vi "Remote.vi"() -> ()   [LabVIEW 2020]
uses:
  LMH-PS4/Private/Type Defs/Indicators/Controller.ctl
  LMH-PS4/Private/Type Defs/Indicators/Square.ctl
  LMH-PS4/Private/Type Defs/Indicators/X.ctl
  LMH-PS4/Private/Type Defs/Indicators/Circle.ctl
  LMH-PS4/Private/Type Defs/Indicators/Triangle.ctl
  LMH-PS4/Private/Type Defs/Indicators/L1.ctl
  LMH-PS4/Private/Type Defs/Indicators/R1.ctl
  LMH-PS4/Private/Type Defs/Indicators/Share.ctl
  LMH-PS4/Private/Type Defs/Indicators/Options.ctl
  LMH-PS4/Private/Type Defs/Indicators/PS.ctl
  LMH-PS4/Private/Type Defs/Indicators/Pad_Button.ctl
  LMH-PS4/Private/Type Defs/Indicators/Dpad.ctl
  LMH-PS4/Private/Type Defs/Indicators/Slider.ctl
  <vilib>/Platform/TimedLoop/XDataNode/timing_clust.ctl
  <vilib>/Platform/TimedLoop/XDataNode/nitl_modes.ctl
  <vilib>/Platform/TimedLoop/XDataNode/wakeup.ctl
  <vilib>/CISH Robotics/L4VMX VMXpi/Type Def/VMX Channel Index.ctl
  <vilib>/CISH Robotics/L4VMX TitanQuad/Motor ID.ctl
  <vilib>/CISH Robotics/L4VMX TitanQuad/TitanQuad.lvclass
  <vilib>/CISH Robotics/L4VMX VMXpi/PWM Generator/PWM Generator.lvclass
  <vilib>/platform/TimedLoop/XDataNode/XDataNode.xnode
  <vilib>/ReMiSYS Technology/RemoteToolkit/Receiver/Receiver.lvclass
  LMH-PS4/LMH-PS4.lvlib
  <vilib>/CISH Robotics/L4VMX VMXpi/Power/Power.lvclass
  <vilib>/Platform/TimedLoop/XDataNode/XDNodeRunTimeDep.lvlib
  <vilib>/CISH Robotics/L4VMX VMXpi/L4VMX.lvlib
  <vilib>/CISH Robotics/L4VMX VMXpi/Utilities/Utilities.lvclass
  <vilib>/CISH Robotics/L4VMX VMXpi/Digital Output/Digital Output.lvclass
  <vilib>/CISH Robotics/L4VMX VMXpi/Digital Input/Digital Input.lvclass
panel:
  out "x/y":dbl
  out "Stop0":bool
  out "result":dbl[](array[numeric])
  out "Voltage":sgl
  out "Error Out":errorcluster
  in  "Stop":bool
  out "Received?":bool
  out "PS4 Controller":T1={"Square Button"=FALSE, "X Button"=FALSE, "Circle Button"=FALSE, "Triangle Button"=FALSE, "L1"=FALSE, "R1"=FALSE, "Share Button"=FALSE, "Options Button"=FALSE, "PS Button"=FALSE, "Pad Button"=FALSE, "D-Pad"=5, "L2"=0, "R2"=0, "Thumbstick_Left"={[], []}, "Thumbstick_Right"={[], []}} {"R2" scale=-32768.0..32767.0; "L2" scale=-32768.0..32767.0}
  # "ss"
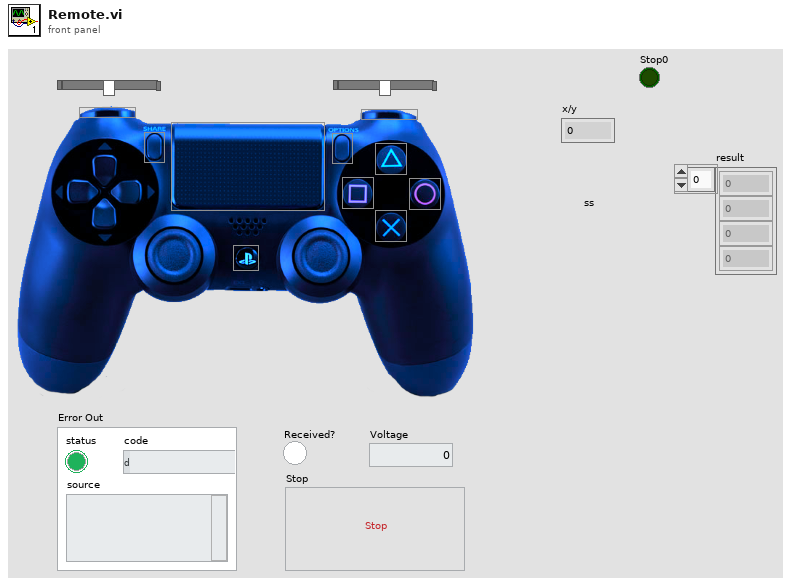
[diagram p1: front panel]
types:
  T1 = typedef "LMH-PS4.lvlib/Controller.ctl" = cluster{"Square Button":T2, "X Button":T3, "Circle Button":T4, "Triangle Button":T5, "L1":T6, "R1":T7, "Share Button":T8, "Options Button":T9, "PS Button":T10, "Pad Button":T11, "D-Pad":T12, "L2":T13, "R2":T13, "Thumbstick_Left":cluster{i32[], i32[]}, "Thumbstick_Right":cluster{i32[], i32[]}}
  T2 = typedef "LMH-PS4.lvlib/Square.ctl" = bool
  T3 = typedef "LMH-PS4.lvlib/X.ctl" = bool
  T4 = typedef "LMH-PS4.lvlib/Circle.ctl" = bool
  T5 = typedef "LMH-PS4.lvlib/Triangle.ctl" = bool
  T6 = typedef "LMH-PS4.lvlib/L1.ctl" = bool
  T7 = typedef "LMH-PS4.lvlib/R1.ctl" = bool
  T8 = typedef "LMH-PS4.lvlib/Share.ctl" = bool
  T9 = typedef "LMH-PS4.lvlib/Options.ctl" = bool
  T10 = typedef "LMH-PS4.lvlib/PS.ctl" = bool
  T11 = typedef "LMH-PS4.lvlib/Pad_Button.ctl" = bool
  T12 = typedef "LMH-PS4.lvlib/Dpad.ctl" = u16
  T13 = typedef "LMH-PS4.lvlib/Slider.ctl" = i32
  T14 = typedef "L4VMX.lvlib/VMX Channel Index.ctl" = enum16{"0", "1", "2", "3", "4", "5", "6", "7", "8", "9", "10", "11", "12", "13", "14", "15", "16", "17", "18", "19", "20", "21", "22", "23", "24", "25", "26", "27", "28", "29", "30", "31", "32", "33"}
  T15 = typedef "TitanQuad.lvlib/TitanQuad.lvclass/Motor ID.ctl" = enum16{"M0", "M1", "M2", "M3"}
  T16 = typedef "XDNodeRunTimeDep.lvlib/timing_clust.ctl" = cluster{"Expected End [f-1]":u64, "Actual End [f-1]":u64, "Finished Late? [f-1]":bool, "Expected End [i-1]":u64, "Actual End [i-1]":u64, "Finished Late? [i-1]":bool, "Expected Start [i]":u64, "Actual Start [i]":u64, "Expected Start [f]":u64, "Actual Start [f]":u64, "Source Name":string, "Structure Name":string, "Period":i64, "Deadline":i64, "Offset":i64, "Start":i64, "Priority":i32, "Timeout":i32, "Mode":T17, "Wakeup Reason":T18, "Error":errorcluster, "Source Type":string, "Secondary Source Type":string, "Global End Time":u64, "Global Start Time":u64, "Frame Duration":u64, "Iteration Duration":u64, "Assigned CPU":i32, "I/O Scan Engine Mode":u32}
  T17 = typedef "XDNodeRunTimeDep.lvlib/nitl_modes.ctl" = enum32{"No Change", "Process missed periods, maintain original phase", "Discard missed periods, maintain original phase", "Process missed periods, ignore original phase", "Discard missed periods, ignore original phase"}
  T18 = typedef "XDNodeRunTimeDep.lvlib/wakeup.ctl" = enum32{"Normal", "Aborted", "Asynchronous wakeup", "Timing source error", "Timed loop error", "Timeout"}
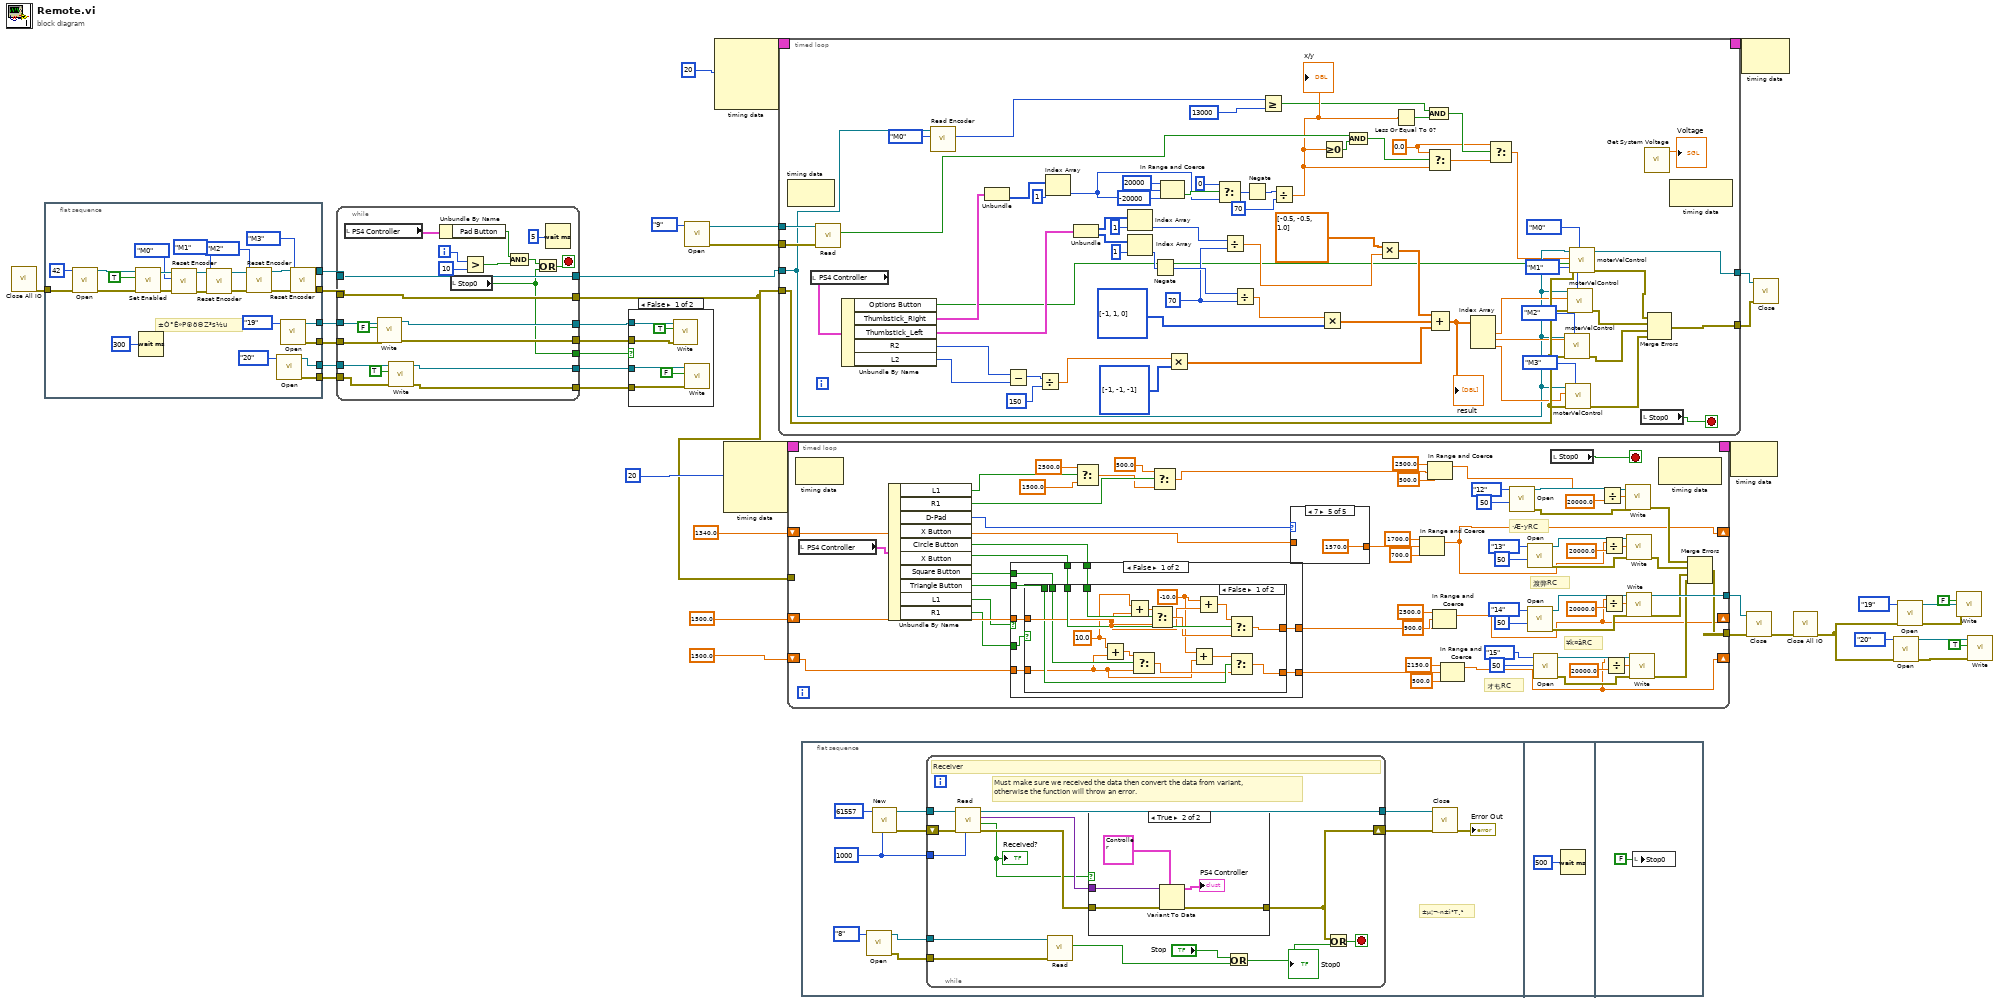
[diagram p0: block diagram]
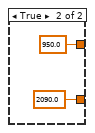
[diagram p3: hidden frame]
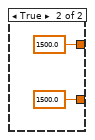
[diagram p4: hidden frame]
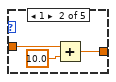
[diagram p6: hidden frame]
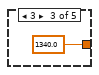
[diagram p7: hidden frame]
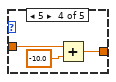
[diagram p8: hidden frame]
diagram:
  n1 = call <vilib>:"Close All IO.vi"() -> ("Error Out"=w15:errorcluster)  [unwired: 11 in]
  n2 = flat-sequence {
    tunnel: [w56] -> w24
    tunnel: [w55] -> w25
    tunnel: [w45] -> w23
    tunnel: [w44] -> w22
    tunnel: [w43] -> w21
    tunnel: [w42] -> w20
    tunnel: w15 -> [w41]
    frame #0 {
      # "±Ò°Ê»P®õ©Z³s½u"
      n3 = call <vilib>:"Open.vi"("Error In"=w41, "Titan ID (42)"=u8 42) -> ("Error Out"=w65:errorcluster, "TitanQuad Object"=w66:refnum<class "TitanQuad.lvclass">)  [unwired: 8 in]
      n4 = call <vilib>:"Set Enabled.vi"("Error In"=w65, "Enable"=TRUE, "TitanQuad Object"=w66) -> ("Error Out"=w52:errorcluster, "TitanQuad Object"=w53:refnum<class "TitanQuad.lvclass">)  [unwired: 7 in]
      n5 = Wait (ms)(milliseconds to wait=u32 300) -> ()  [unwired: 1 out]
      n6 = call <vilib>:"Reset Encoder.vi"("Error In"=w52, "Motor ID"=Motor_ID."M0", "TitanQuad Object"=w53) -> ("Error Out"=w62:errorcluster, "TitanQuad Object"=w61:refnum<class "TitanQuad.lvclass">)  [unwired: 7 in]
      n7 = call <vilib>:"Reset Encoder.vi"("Error In"=w62, "Motor ID"=Motor_ID."M1", "TitanQuad Object"=w61) -> ("Error Out"=w59:errorcluster, "TitanQuad Object"=w60:refnum<class "TitanQuad.lvclass">)  [unwired: 7 in]
      n8 = call <vilib>:"Reset Encoder.vi"("Error In"=w59, "Motor ID"=Motor_ID."M2", "TitanQuad Object"=w60) -> ("Error Out"=w57:errorcluster, "TitanQuad Object"=w58:refnum<class "TitanQuad.lvclass">)  [unwired: 7 in]
      n9 = call <vilib>:"Open.vi"("VMX Channel Index"=VMX_Channel_Index."20") -> ("Error Out"=w42:errorcluster, "Digital Output Object"=w43:refnum<class "Digital Output.lvclass">)  [unwired: 9 in]
      n10 = call <vilib>:"Open.vi"("VMX Channel Index"=VMX_Channel_Index."19") -> ("Error Out"=w44:errorcluster, "Digital Output Object"=w45:refnum<class "Digital Output.lvclass">)  [unwired: 9 in]
      n11 = call <vilib>:"Reset Encoder.vi"("Error In"=w57, "Motor ID"=Motor_ID."M3", "TitanQuad Object"=w58) -> ("Error Out"=w56:errorcluster, "TitanQuad Object"=w55:refnum<class "TitanQuad.lvclass">)  [unwired: 7 in]
    }
  }
  n12 = while {
    tunnel: [w87] -> w26
    tunnel: w25 -> [w87]
    tunnel: [w86] -> w1
    tunnel: w24 -> [w86]
    tunnel: w23 -> [w79]
    tunnel: w22 -> [w78]
    tunnel: w21 -> [w77]
    tunnel: w20 -> [w76]
    tunnel: [w75] -> w19
    tunnel: [w74] -> w18
    tunnel: [w73] -> w17
    tunnel: [w72] -> w16
    tunnel: [w67] -> w5
    i -> [w82]
    stop <- w68 stop-if-true
    n13 = local read "PS4 Controller"() -> (w85:T1)
    n14 = call <vilib>:"Write.vi"("Error In"=w78, "Value"=FALSE, "Digital Output Object"=w79) -> ("Error Out"=w74:errorcluster, "Digital Output Object"=w75:refnum<class "Digital Output.lvclass">)  [unwired: 7 in]
    n15 = call <vilib>:"Write.vi"("Error In"=w76, "Value"=TRUE, "Digital Output Object"=w77) -> ("Error Out"=w72:errorcluster, "Digital Output Object"=w73:refnum<class "Digital Output.lvclass">)  [unwired: 7 in]
    n16 = Unbundle By Name(w85) -> ("Pad Button"=w83:T11)
    n17 = local read "Stop0"() -> (w67:bool)
    n18 = Greater?(x=w82, y=10) -> (0:w80:bool)
    n19 = And(x=w83, y=w80) -> (x .and. y?=w69:T11)
    n20 = Or(x=w69, y=w67) -> (x .or. y?=w68:T11)
    n21 = Wait (ms)(milliseconds to wait=u32 5) -> ()  [unwired: 1 out]
  }
  n22 = case shown="False" w5 {
    tunnel: w19 -> [w93 _]
    tunnel: w18 -> [w92 _]
    tunnel: w17 -> [w91 _]
    tunnel: w16 -> [w90 _]
    frame False {
      n23 = call <vilib>:"Write.vi"("Error In"=w92, "Value"=TRUE, "Digital Output Object"=w93) -> ()  [unwired: 7 in, 2 out]
      n24 = call <vilib>:"Write.vi"("Error In"=w90, "Value"=FALSE, "Digital Output Object"=w91) -> ()  [unwired: 7 in, 2 out]
    }
    frame True {
    }
  }
  n25 = call <vilib>:"Open.vi"("VMX Channel Index"=VMX_Channel_Index."9") -> ("Error Out"=w3:errorcluster, "Digital Input Object"=w2:refnum<class "Digital Input.lvclass">)  [unwired: 9 in]
  n26 = node-c288(i64 20 ("Period")) -> (w40:T16)  [unwired: 3 in]
  n27 = node-c288(i64 20 ("Period")) -> (w35:T16)  [unwired: 3 in]
  n28 = timed-loop {
    timing: w40 -> [_]
    timing-out: [_] -> w39
    tunnel: w26 -> [w107]
    tunnel: w1 -> [w127]
    tunnel: [w159] -> w37
    tunnel: [w131] -> w36
    tunnel: w3 -> [w110]
    tunnel: w2 -> [w109]
    stop <- w161 stop-if-true
    w97 = 0.0 ("t")
    w143 = 70 ("y")
    n29 = node-c288() -> ()  [unwired: 1 in, 1 out]
    n30 = local read "PS4 Controller"() -> (w158:T1)
    n31 = call <vilib>:"Read.vi"("Error In"=w110, "Digital Input Object"=w109) -> ("Value"=w104:bool)  [unwired: 7 in, 2 out]
    n32 = Unbundle By Name(w158) -> ("Options Button"=w108:T9, "Thumbstick_Right"=w117:cluster{i32[], i32[]}, "Thumbstick_Left"=w118:cluster{i32[], i32[]}, "R2"=w157:T13, "L2"=w156:T13)
    n33 = call <vilib>:"Read Encoder.vi"("Motor ID"=Motor_ID."M0", "TitanQuad Object"=w107) -> ("Counter Value"=w96:i32)  [unwired: 7 in, 2 out]
    n34 = Unbundle(w117) -> (w154:i32[])  [unwired: 1 out]
    n35 = Subtract(x=w157, y=w156) -> (x-y=w141:T13)
    n36 = Divide(x=w141, y=150) -> (x/y=w140:dbl)
    n37 = Index Array(array=w154, index=1) -> (element=w112:i32)
    n38 = Unbundle(w118) -> (w152:i32[], w151:i32[])
    n39 = Index Array(array=w152, index=1) -> (element=w139:i32)
    n40 = Index Array(array=w151, index=1) -> (element=w145:i32)
    n41 = Negate(x=w145) -> (-x=w144:i32)
    n42 = In Range and Coerce(upper limit=20000, x=w112, lower limit=-20000) -> (In Range?=w114:bool)  [unwired: 1 out]
    n43 = Multiply(x=w140, y=i32[] [-1, -1, -1]) -> (x*y=w155:dbl[])
    n44 = Select(t=0, s=w114, f=w112) -> (s? t:f=w111:i32)
    n45 = Divide(x=w139, y=w143) -> (x/y=w119:dbl)
    n46 = Divide(x=w144, y=w143) -> (x/y=w138:dbl)
    n47 = Negate(x=w111) -> (-x=w147:i32)
    n48 = Greater Or Equal?(x=w96, y=13000) -> (x >= y?=w94:bool)
    n49 = Divide(x=w147, y=70) -> (x/y=w100:dbl)
    "x/y" <- w100
    n50 = Multiply(x=w138, y=i32[] [-1, 1, 0]) -> (x*y=w134:dbl[])
    n51 = Greater Or Equal To 0?(x=w100) -> (x >= 0?=w105:bool)
    n52 = And(x=w104, y=w105) -> (x .and. y?=w103:bool)
    n53 = Multiply(x=dbl[] [-0.5, -0.5, 1.0], y=w119) -> (x*y=w135:dbl[])
    n54 = Less Or Equal To 0?(x=w100) -> (x <= 0?=w99:bool)
    n55 = And(x=w94, y=w99) -> (x .and. y?=w98:bool)
    n56 = Select(t=w97, s=w103, f=w100) -> (s? t:f=w102:dbl)
    n57 = Compound Arithmetic op=ADD(w135, w134, w155) -> (w153:dbl[])
    "result" <- w153
    n58 = Index Array(array=w153) -> (element #1=w126:dbl, element #2=w122:dbl, element #3=w121:dbl)  [unwired: 3 in]
    n59 = Select(t=w97, s=w98, f=w102) -> (s? t:f=w101:dbl)
    n60 = call "moterVelControl.vi"("Motor ID"=Motor_ID."M2", "error in"=w127, "Speed (deg/s)"=w122, "TitanQuad Object"=w107) -> ("error out"=w129:errorcluster)  [unwired: 6 in, 1 out]
    n61 = call "moterVelControl.vi"("Motor ID"=Motor_ID."M3", "error in"=w127, "Speed (deg/s)"=w121, "TitanQuad Object"=w107) -> ("error out"=w130:errorcluster)  [unwired: 6 in, 1 out]
    n62 = call "moterVelControl.vi"("Motor ID"=Motor_ID."M1", "error in"=w127, "Speed (deg/s)"=w126, "TitanQuad Object"=w107) -> ("error out"=w128:errorcluster)  [unwired: 6 in, 1 out]
    n63 = call "moterVelControl.vi"("Motor ID"=Motor_ID."M0", "error in"=w127, "reset?"=w108, "Speed (deg/s)"=w101, "TitanQuad Object"=w107) -> ("error out"=w132:errorcluster, "TitanQuad Object 2"=w131:refnum<class "TitanQuad.lvclass">)  [unwired: 5 in]
    n64 = local read "Stop0"() -> (w161:bool)
    n65 = call <vilib>:"Get System Voltage.vi"() -> ("Voltage"=→"Voltage":sgl)  [unwired: 10 in, 1 out]
    n66 = Merge Errors(w132, w128, w129, w130) -> (w159:errorcluster)
    n67 = node-c288() -> ()  [unwired: 1 in, 1 out]
  }
  n68 = timed-loop {
    timing: w35 -> [_]
    timing-out: [_] -> w34
    tunnel: [w212] -> w31
    tunnel: [w223] -> w30
    shift-right: [w187] -> _
    shift-left: 1500.0 ("y") -> [w192]
    shift-right: [w183] -> _
    shift-left: 1500.0 ("y") -> [w189]
    shift-right: [w174] -> _
    shift-left: 1340.0 ("y") -> [w180]
    tunnel: w1 -> [_]
    stop <- w227 stop-if-true
    # "オもRC"
    # "¥k¤âRC"
    # "渡弊RC"
    # "·Æ­yRC"
    n69 = node-c288() -> ()  [unwired: 1 in, 1 out]
    n70 = local read "PS4 Controller"() -> (w226:T1)
    n71 = Unbundle By Name(w226) -> ("L1"=w170:T6, "R1"=w169:T7, "D-Pad"=w195:T12, "Circle Button"=w194:T4, "X Button"=w193:T3, "Square Button"=w191:T2, "Triangle Button"=w190:T5, "L1"=w172:T6, "R1"=w171:T7)  [unwired: 1 out]
    n72 = case shown="False" w172 {
      tunnel: w194 -> [w236 _]
      tunnel: w193 -> [w235 _]
      tunnel: w192 -> [w234 _]
      tunnel: w191 -> [w233 _]
      tunnel: w190 -> [w232 _]
      tunnel: w189 -> [w231 _]
      tunnel: [w230 1500.0 ("y")] -> w188
      tunnel: [w229 1500.0 ("y")] -> w184
      tunnel: w171 -> [w228 _]
      frame False {
        n73 = case shown="False" w228 {
          tunnel: w236 -> [w252 _]
          tunnel: w235 -> [w251 _]
          tunnel: w234 -> [w248 _]
          tunnel: w233 -> [w246 _]
          tunnel: w232 -> [w245 _]
          tunnel: w231 -> [w242 _]
          tunnel: [w240 950.0 ("y")] -> w230
          tunnel: [w239 2090.0 ("y")] -> w229
          frame False {
            w238 = 10.0 ("x")
            w237 = -10.0 ("x")
            n74 = Add(x=w238, y=w242) -> (x+y=w244:dbl)
            n75 = Add(x=w238, y=w248) -> (x+y=w249:dbl)
            n76 = Select(t=w244, s=w246, f=w242) -> (s? t:f=w243:dbl)
            n77 = Select(t=w249, s=w252, f=w248) -> (s? t:f=w250:dbl)
            n78 = Add(x=w237, y=w242) -> (x+y=w241:dbl)
            n79 = Add(x=w237, y=w248) -> (x+y=w247:dbl)
            n80 = Select(t=w247, s=w251, f=w250) -> (s? t:f=w240:dbl)
            n81 = Select(t=w241, s=w245, f=w243) -> (s? t:f=w239:dbl)
          }
          frame True {
          }
        }
      }
      frame True {
      }
    }
    n82 = Select(t=2500.0, s=w170, f=1500.0 ("lower limit")) -> (s? t:f=w167:dbl)
    n83 = Select(t=500.0, s=w169, f=w167) -> (s? t:f=w164:dbl)
    n84 = case shown="7" w195 {
      tunnel: w180 -> [w257 w260 _ w264 _]
      tunnel: [w257 w258 1340.0 ("y") w262 1570.0 ("y")] -> w175
      frame 0, Default {
      }
      frame 1 {
        n85 = Add(x=w260, y=10.0) -> (x+y=w258:dbl)
      }
      frame 3 {
      }
      frame 5 {
        n86 = Add(x=w264, y=-10.0) -> (x+y=w262:dbl)
      }
      frame 7 {
      }
    }
    n87 = In Range and Coerce(upper limit=1700.0, x=w175, lower limit=700.0) -> (coerced(x)=w174:dbl)  [unwired: 1 out]
    n88 = In Range and Coerce(upper limit=2500.0, x=w164, lower limit=500.0) -> (coerced(x)=w177:dbl)  [unwired: 1 out]
    n89 = In Range and Coerce(upper limit=2500.0, x=w188, lower limit=900.0) -> (coerced(x)=w187:dbl)  [unwired: 1 out]
    n90 = In Range and Coerce(upper limit=2150.0, x=w184, lower limit=500.0) -> (coerced(x)=w183:dbl)  [unwired: 1 out]
    n91 = call <vilib>:"Open.vi"("Frequency(Hz)"=u32 50, "VMX Channel Index"=VMX_Channel_Index."12") -> ("Error Out"=w202:errorcluster, "PWM Generator Object"=w203:refnum<class "PWM Generator.lvclass">)  [unwired: 8 in]
    n92 = call <vilib>:"Open.vi"("Frequency(Hz)"=u32 50, "VMX Channel Index"=VMX_Channel_Index."13") -> ("Error Out"=w200:errorcluster, "PWM Generator Object"=w201:refnum<class "PWM Generator.lvclass">)  [unwired: 8 in]
    n93 = call <vilib>:"Open.vi"("Frequency(Hz)"=u32 50, "VMX Channel Index"=VMX_Channel_Index."14") -> ("Error Out"=w198:errorcluster, "PWM Generator Object"=w199:refnum<class "PWM Generator.lvclass">)  [unwired: 8 in]
    n94 = call <vilib>:"Open.vi"("Frequency(Hz)"=u32 50, "VMX Channel Index"=VMX_Channel_Index."15") -> ("Error Out"=w196:errorcluster, "PWM Generator Object"=w197:refnum<class "PWM Generator.lvclass">)  [unwired: 8 in]
    n95 = local read "Stop0"() -> (w227:bool)
    n96 = Divide(x=w177, y=20000.0) -> (x/y=w219:dbl)
    n97 = Divide(x=w174, y=20000.0) -> (x/y=w218:dbl)
    n98 = Divide(x=w187, y=20000.0) -> (x/y=w224:dbl)
    n99 = Divide(x=w183, y=20000.0) -> (x/y=w222:dbl)
    n100 = call <vilib>:"Write.vi"("Error In"=w202, "Duty Cycle(0~1)"=w219, "PWM Generator Object"=w203) -> ("Error Out"=w216:errorcluster)  [unwired: 7 in, 1 out]
    n101 = call <vilib>:"Write.vi"("Error In"=w200, "Duty Cycle(0~1)"=w218, "PWM Generator Object"=w201) -> ("Error Out"=w215:errorcluster)  [unwired: 7 in, 1 out]
    n102 = call <vilib>:"Write.vi"("Error In"=w198, "Duty Cycle(0~1)"=w224, "PWM Generator Object"=w199) -> ("Error Out"=w214:errorcluster, "PWM Generator Object"=w223:refnum<class "PWM Generator.lvclass">)  [unwired: 7 in]
    n103 = call <vilib>:"Write.vi"("Error In"=w196, "Duty Cycle(0~1)"=w222, "PWM Generator Object"=w197) -> ("Error Out"=w213:errorcluster)  [unwired: 7 in, 1 out]
    n104 = node-c288() -> ()  [unwired: 1 in, 1 out]
    n105 = Merge Errors(w216, w215, w214, w213) -> (w212:errorcluster)
  }
  n106 = flat-sequence {
    frame #0 {
      w273 = 1000 ("Timeout ms (25000)")
      # "±µ¦¬·n±ì°T¸¹"
      n107 = call <vilib>:"Open.vi"("VMX Channel Index"=VMX_Channel_Index."8") -> ("Error Out"=w268:errorcluster, "Digital Input Object"=w269:refnum<class "Digital Input.lvclass">)  [unwired: 9 in]
      n108 = call <vilib>:"New.vi"("Timeout ms (25000)"=w273, "Port (61557)"=u16 61557) -> ("Error Out"=w277:errorcluster, "Receiver Ref."=w276:refnum<class "Receiver.lvclass">)  [unwired: 8 in]
      n109 = while {
        shift-right: [w284] -> w275
        shift-left: w277 -> [w291]
        tunnel: w276 -> [w290]
        tunnel: [w289] -> w274
        tunnel: w273 -> [w288]
        tunnel: w269 -> [w282]
        tunnel: w268 -> [w281]
        stop <- w287 stop-if-true
        # "Must make sure we received the data then convert the data from variant,\notherwise the function will throw an error."
        # "Receiver"
        n110 = call <vilib>:"Read.vi"("Timeout ms (1000)"=w288, "Error In"=w291, "Receiver Ref."=w290) -> ("Error Out"=w286:errorcluster, "Received?"=w283:bool, "Value"=w285:variant, "Receiver Ref."=w289:refnum<class "Receiver.lvclass">)  [unwired: 5 in]
        "Received?" <- w283
        n111 = call <vilib>:"Read.vi"("Error In"=w281, "Digital Input Object"=w282) -> ("Value"=w280:bool)  [unwired: 7 in, 2 out]
        n112 = case shown="True" w283 {
          tunnel: w286 -> [w292 w297]
          tunnel: w285 -> [_ w296]
          tunnel: [w292 w295] -> w284
          frame False {
          }
          frame True {
            n113 = Variant To Data(error in=w297, type=T1 {"Square Button"=FALSE, "X Button"=FALSE, "Circle Button"=FALSE, "Triangle Button"=FALSE, "L1"=FALSE, "R1"=FALSE, "Share Button"=FALSE, "Options Button"=FALSE, "PS Button"=FALSE, "Pad Button"=FALSE, "D-Pad"=0, "L2"=-32768, "R2"=-32768, "Thumbstick_Left"={[0, 0], [0, 0]}, "Thumbstick_Right"={[0, 0], [0, 0]}} ("PS4 Controller"), Variant=w296) -> (data=→"PS4 Controller":T1, error out=w295:errorcluster)
          }
        }
        n114 = Or(x="Stop", y=w280) -> (x .or. y?=w278:bool)
        "Stop0" <- w278
        n115 = Or(x=w284, y=w278) -> (x .or. y?=w287:bool)
      }
      n116 = call <vilib>:"Close.vi"("Error In"=w275, "Receiver Ref."=w274) -> ("Error Out"=→"Error Out":errorcluster)  [unwired: 9 in]
    }
    frame #1 {
      n117 = Wait (ms)(milliseconds to wait=u32 500) -> ()  [unwired: 1 out]
    }
    frame #2 {
      n118 = local write "Stop0"(FALSE ("Stop")) -> ()
    }
  }
  n119 = node-c288(w34) -> ()  [unwired: 1 out]
  n120 = node-c288(w39) -> ()  [unwired: 1 out]
  n121 = call <vilib>:"Close.vi"("Error In"=w31, "PWM Generator Object"=w30) -> ("Error Out"=w32:errorcluster)  [unwired: 9 in]
  n122 = call <vilib>:"Close.vi"("Error In"=w37, "TitanQuad Object"=w36) -> ()  [unwired: 9 in, 1 out]
  n123 = call <vilib>:"Close All IO.vi"("Error In"=w32) -> ("Error Out"=w10:errorcluster)  [unwired: 10 in]
  n124 = call <vilib>:"Open.vi"("Error In"=w10, "VMX Channel Index"=VMX_Channel_Index."20") -> ("Error Out"=w8:errorcluster, "Digital Output Object"=w9:refnum<class "Digital Output.lvclass">)  [unwired: 8 in]
  n125 = call <vilib>:"Open.vi"("Error In"=w10, "VMX Channel Index"=VMX_Channel_Index."19") -> ("Error Out"=w6:errorcluster, "Digital Output Object"=w7:refnum<class "Digital Output.lvclass">)  [unwired: 8 in]
  n126 = call <vilib>:"Write.vi"("Error In"=w6, "Value"=FALSE, "Digital Output Object"=w7) -> ()  [unwired: 7 in, 2 out]
  n127 = call <vilib>:"Write.vi"("Error In"=w8, "Value"=TRUE, "Digital Output Object"=w9) -> ()  [unwired: 7 in, 2 out]
